vi "nntcpsendrecv.vi"(8 "error in (no error)":errorcluster, 10 "String":string, 11 "TCP Network Connection in":refnum<k5>) -> (0 "error out":errorcluster, 2 "data out":string, 3 "TCP Network Connection out":refnum<k5>)   [LabVIEW 2018, in "nn.lvlib"]
uses:
  nn.lvlib
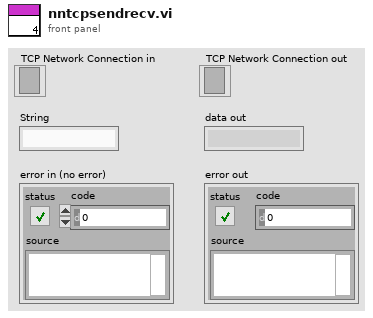
[diagram p1: front panel]
types:
  T1 = enum16{"Standard", "Buffered", "CRLF", "Immediate"}
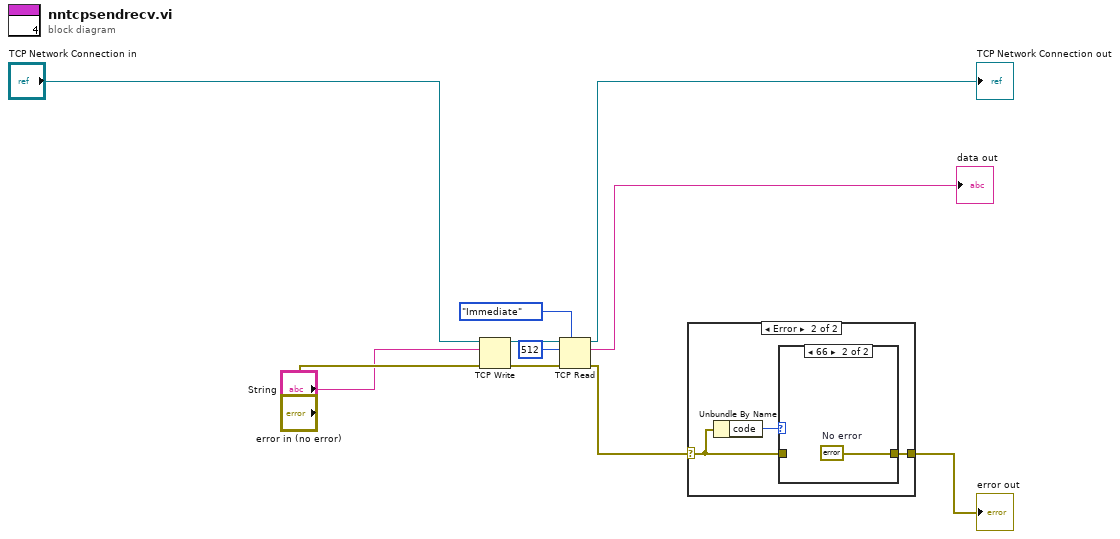
[diagram p0: block diagram]
diagram:
  n1 = TCP Write(connection ID="TCP Network Connection in", data in="String", error in (no error)="error in (no error)") -> (connection ID out=w2:refnum<k5>, error out=w1:errorcluster)  [unwired: 1 in, 1 out]
  n2 = TCP Read(connection ID=w2, bytes to read=512, error in (no error)=w1, 7:T1."Immediate" ("mode (standard)")) -> (connection ID out=→"TCP Network Connection out":refnum<k5>, data out=→"data out":string, error out=w9:errorcluster)  [unwired: 1 in]
  n3 = case shown="Error" w9 {
    selector: w9 -> [w12 w14]
    tunnel: [w12 w13] -> w10
    frame No Error {
    }
    frame Error {
      n4 = Unbundle By Name(w14) -> ("code"=w15:i32)
      n5 = case shown="66" w15 {
        tunnel: w14 -> [w16 _]
        tunnel: [w16 w17] -> w13
        frame Default {
        }
        frame 66 {
          w17 = errorcluster {"status"=FALSE, "code"=0, "source"=""}  # No error
        }
      }
    }
  }
  "error out" <- w10
